vi "GetPrimeConfigKeys.vi"() -> (3 "Prime Names":T1)   [LabVIEW 2022 SP3]
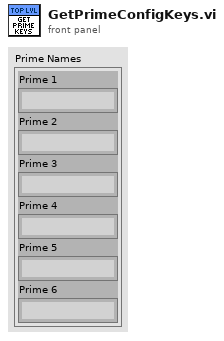
[diagram p1: front panel]
types:
  T1 = cluster{"Prime 1":string, "Prime 2":string, "Prime 3":string, "Prime 4":string, "Prime 5":string, "Prime 6":string}
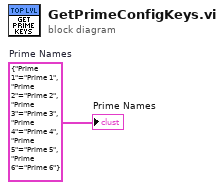
[diagram p0: block diagram]
diagram:
  w1 = T1 {"Prime 1"="Prime 1", "Prime 2"="Prime 2", "Prime 3"="Prime 3", "Prime 4"="Prime 4", "Prime 5"="Prime 5", "Prime 6"="Prime 6"}  # Prime Names
  "Prime Names" <- w1
